vi "PFI-28000-Card_Destroy.vi"(0 "PFI-28000-Card in":refnum<class "PFI-28000-Card.lvclass">, 11 "error in (no error)":errorcluster) -> (15 "error out":errorcluster)   [LabVIEW 2017, in "PFI-28000-Card.lvclass"]
uses:
  PFI-28000-Card.lvclass
  PFI-28000-Card.lvclass/PFI-28000-Card.ctl
  Channel/PFI-28000-Channel.lvclass
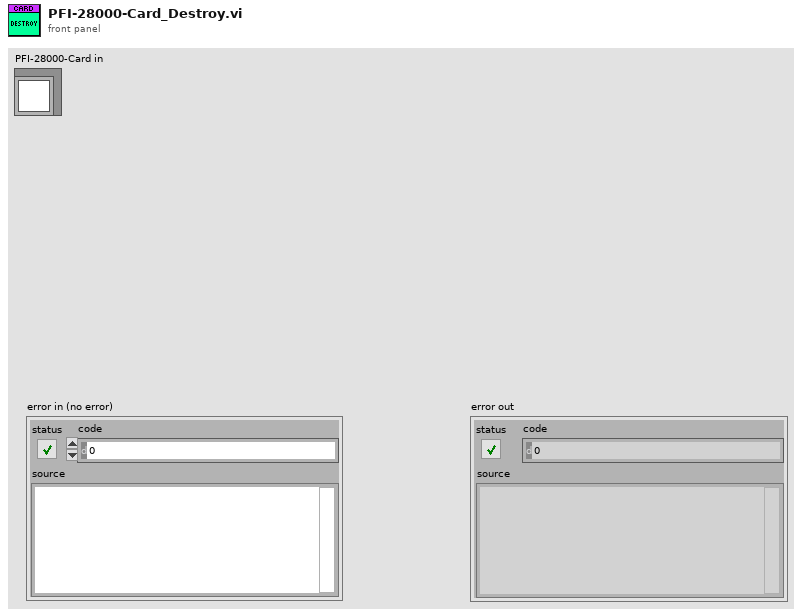
[diagram p1: front panel]
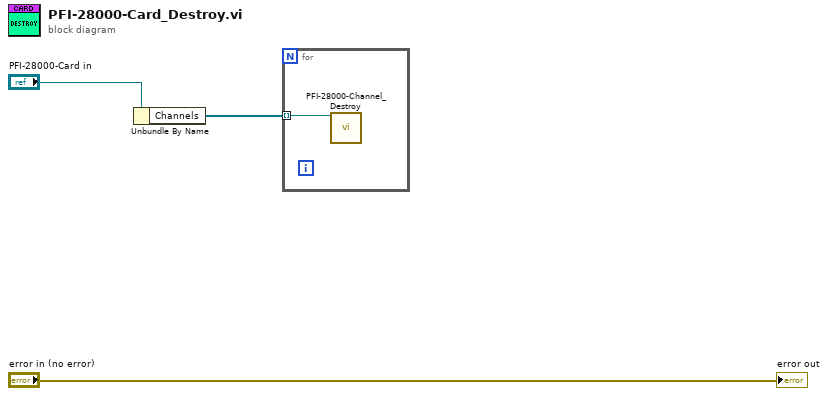
[diagram p0: block diagram]
diagram:
  n1 = Unbundle By Name("PFI-28000-Card in") -> ("Channels"=w1:refnum<class "PFI-28000-Channel.lvclass">[])
  n2 = for {
    tunnel: w1 -> [w4] mode=indexing
    n3 = call-dynamic "PFI-28000-Channel_Destroy.vi"("PFI-28000-Channel in"=w4) -> ()  [unwired: 14 in, 1 out]
  }
  "error out" <- "error in (no error)"
